vi "Detekce_vzestupne.vi"(3 "dt 2":dbl format="%#_13g", 4 "array":dbl[](array[numeric])) -> (0 "Pole indexu pruchodu nulou":i32[](array[numeric]), 1 "Numeric":dbl)   [LabVIEW 2019]
panel:
  out "Boolean":bool
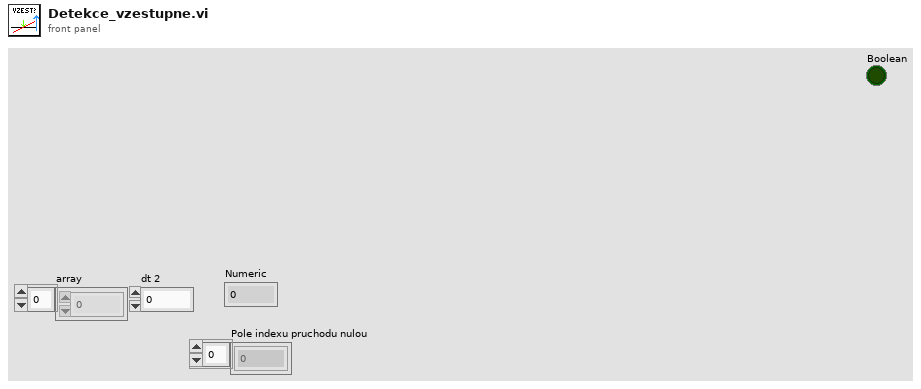
[diagram p1: front panel]
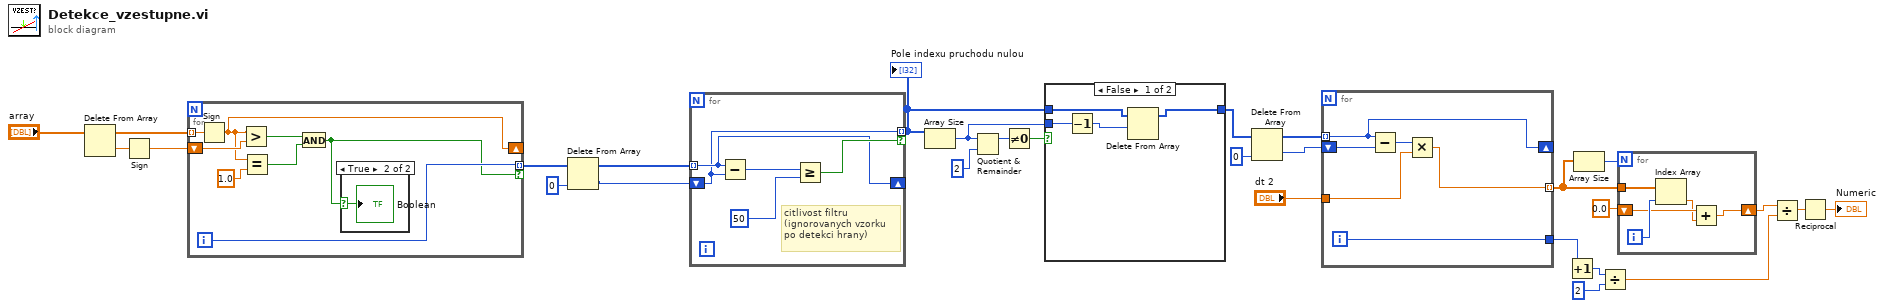
[diagram p0: block diagram]
diagram:
  n1 = Delete From Array(array="array") -> (deleted portion=w26:dbl, array with subset deleted=w28:dbl[])  [unwired: 2 in]
  n2 = Sign(1:w26) -> (0:w25:dbl)
  n3 = for {
    tunnel: w28 -> [w36] mode=indexing
    shift-right: [w32] -> _
    shift-left: w25 -> [w34]
    tunnel: [w35] -> w4 mode=indexing if=w29
    i -> [w35]
    n4 = Sign(1:w36) -> (0:w32:dbl)
    n5 = Greater?(x=w32, y=w34) -> (0:w33:bool)
    n6 = Equal?(x=w32, y=1.0) -> (x = y?=w30:bool)
    n7 = And(x=w33, y=w30) -> (x .and. y?=w29:bool)
    n8 = case shown="True" w29 {
      selector: w29 -> [_ w37]
      frame False {
      }
      frame True {
        "Boolean" <- w37
      }
    }
  }
  n9 = Delete From Array(array=w4, index=0) -> (deleted portion=w1:i32, array with subset deleted=w3:i32[])  [unwired: 1 in]
  n10 = for {
    tunnel: w3 -> [w39] mode=indexing
    shift-right: [w39] -> _
    shift-left: w1 -> [w38]
    tunnel: [w38] -> w17 mode=indexing if=w40
    # "citlivost filtru\n(ignorovanych vzorku\npo detekci hrany)"
    n11 = Subtract(x=w39, y=w38) -> (x-y=w42:i32)
    n12 = Greater Or Equal?(x=w42, y=50 ("Citlivost vypoctu frekvence")) -> (x >= y?=w40:bool)
  }
  "Pole indexu pruchodu nulou" <- w17
  n13 = Array Size(array=w17) -> (size(s)=w15:i32)
  n14 = Quotient & Remainder(x=w15, y=2) -> (x-y*floor(x/y)=w19:i32)  [unwired: 1 out]
  n15 = Not Equal To 0?(x=w19) -> (x != 0?=w18:bool)
  n16 = case shown="False" w18 {
    tunnel: w17 -> [w46 w47]
    tunnel: [w43 w47] -> w16
    tunnel: w15 -> [w45 _]
    frame False {
      n17 = Decrement(x=w45) -> (x-1=w44:i32)
      n18 = Delete From Array(array=w46, length=w44) -> (array with subset deleted=w43:i32[])  [unwired: 1 in, 1 out]
    }
    frame True {
    }
  }
  n19 = Delete From Array(array=w16, index=0) -> (deleted portion=w23:i32, array with subset deleted=w24:i32[])  [unwired: 1 in]
  n20 = for {
    tunnel: w24 -> [w50] mode=indexing
    shift-right: [w50] -> _
    shift-left: w23 -> [w53]
    tunnel: "dt 2" -> [w52]
    tunnel: [w49] -> w21
    tunnel: [w48] -> w13 mode=indexing
    i -> [w49]
    n21 = Subtract(x=w50, y=w53) -> (x-y=w51:i32)
    n22 = Multiply(x=w51, y=w52) -> (x*y=w48:dbl)
  }
  n23 = Increment(x=w21) -> (x+1=w10:i32)
  n24 = Array Size(array=w13) -> (size(s)=w12:i32)
  n25 = Divide(x=w10, y=2) -> (x/y=w8:dbl)
  n26 = for {
    N: w12 -> [_]
    tunnel: w13 -> [w58]
    shift-right: [w54] -> w7
    shift-left: 0.0 -> [w56]
    i -> [w57]
    n27 = Index Array(array=w58, index=w57) -> (element=w55:dbl)
    n28 = Add(x=w56, y=w55) -> (x+y=w54:dbl)
  }
  n29 = Divide(x=w7, y=w8) -> (x/y=w6:dbl)
  n30 = Reciprocal(x=w6) -> (1/x=→"Numeric":dbl)
